vi "Send Value Update.vi"(8 "error in (no error)":errorcluster, 9 "Value":variant, 10 "Datum Name":string, 11 "IViewModel in":refnum<class "IViewModel.lvclass">) -> (0 "error out":errorcluster)   [LabVIEW 2015, in "IViewModel.lvlib" / "IViewModel.lvclass"]
uses:
  IViewModel.lvclass
  <vilib>/ActorFramework/Actor/Actor.lvclass/Actor.ctl
  <vilib>/ActorFramework/Message Enqueuer/Message Enqueuer.lvclass/Message Enqueuer.ctl
  IViewModel.lvclass/IViewModel.ctl
  IMediator/PublishRequest/PublishRequest.lvclass/PublishRequest.ctl
  AbstractMessages/PreAddressedMsg/PreAddressedMsg.lvclass/PreAddressedMsg.ctl
  IMediator/IMediator Messages/Publish Msg/Publish Msg.lvclass/Publish Msg.ctl
  IMediator/IMediator Messages/Publish Msg/Send Pre-Addressed Publish.vi
  IObserver/IObserver/Read Unique ID.vi
  IMediator/PublishRequest/Pack Publish Request.vi
  <vilib>/ActorFramework/Message Enqueuer/Enqueue.vi
  AbstractMessages/PreAddressedMsg/Read Return Address.vi
  <vilib>/ActorFramework/Actor/Read Self Enqueuer.vi
  <vilib>/ActorFramework/Message Enqueuer/Init from Existing Queue.vi
  <vilib>/ActorFramework/Message Priority Queue/Priority Enqueue.vi
  IMediator/PublishRequest/PublishRequest.lvclass
  <vilib>/ActorFramework/Message Enqueuer/Message Enqueuer.lvclass
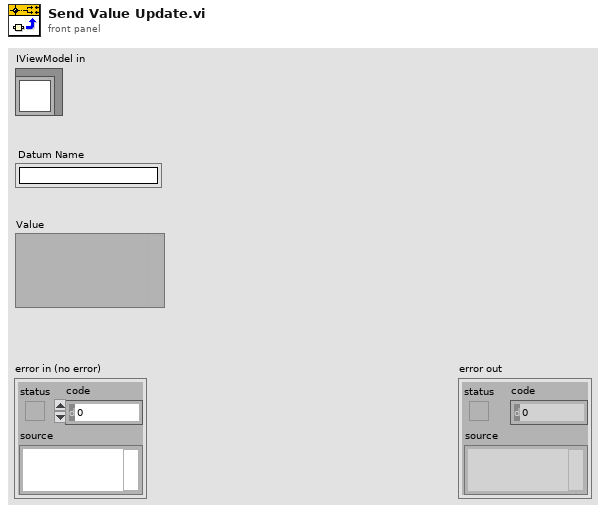
[diagram p1: front panel]
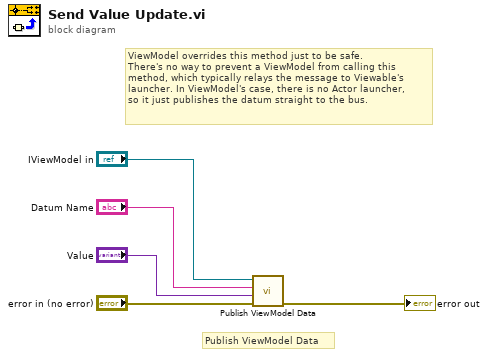
[diagram p0: block diagram]
diagram:
  # "ViewModel overrides this method just to be safe.\nThere's no way to prevent a ViewModel from calling this\nmethod, which typically relays the message to Viewable's\nlauncher. In ViewModel's case, there is no Actor launcher,\nso it just publishes the datum straight to the bus."
  # "Publish ViewModel Data"
  n1 = call "Publish ViewModel Data.vi"("error in (no error)"="error in (no error)", "Data to Publish"="Value", "Datum Name"="Datum Name", "IViewModel In"="IViewModel in") -> ("error out"=→"error out":errorcluster)  [unwired: 6 in, 1 out]
